vi "Overlays.vi"(0 "Image In":T2, 5 "FullArray":dbl[][](array[numeric]), 7 "SelectedGoalSubarray":dbl[](array[numeric]), 9 "ProjectedPosition":cluster{dbl, dbl}, 11 "Enabled Overlay":T3, 13 "Pitch":T1) -> (4 "Image Out":T2)   [LabVIEW 2012]
uses:
  <vilib>/vision/Image Controls.llb/IMAQ Image.ctl
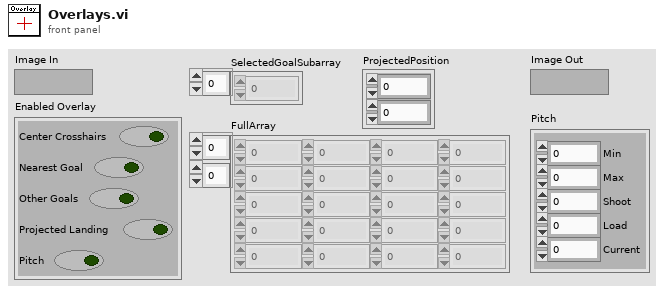
[diagram p1: front panel]
types:
  T1 = cluster{"Min":dbl, "Max":dbl, "Shoot":dbl, "Load":dbl, "Current":dbl}
  T2 = typedef "IMAQ Image.ctl" = refnum<image>
  T3 = cluster{"Center Crosshairs":bool, "Nearest Goal":bool, "Other Goals":bool, "Projected Landing":bool, "Pitch":bool}
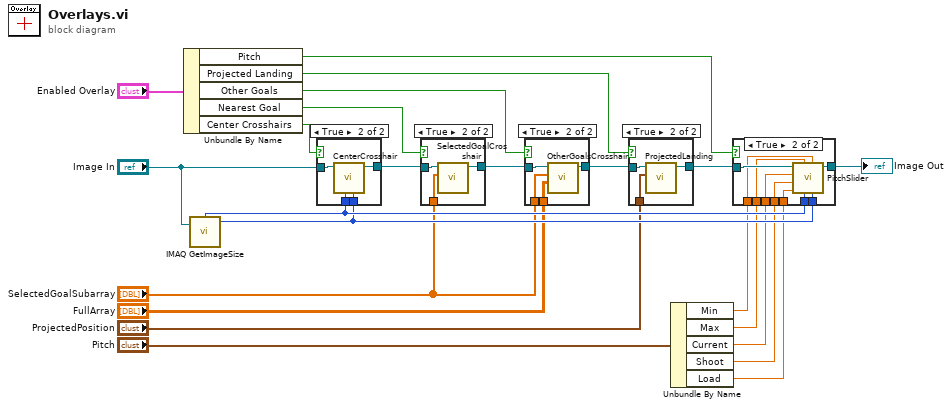
[diagram p0: block diagram]
diagram:
  n1 = Unbundle By Name("Enabled Overlay") -> ("Pitch"=w16:bool, "Projected Landing"=w17:bool, "Other Goals"=w18:bool, "Nearest Goal"=w20:bool, "Center Crosshairs"=w22:bool)
  n2 = call "IMAQ GetImageSize"("Image"="Image In") -> ("Y Resolution"=w10:i32, "X Resolution"=w11:i32)  [unwired: 3 in, 1 out]
  n3 = case shown="True" w22 {
    tunnel: "Image In" -> [w24 w28]
    tunnel: [w24 w27] -> w21
    tunnel: w11 -> [_ w26]
    tunnel: w10 -> [_ w25]
    frame False {
    }
    frame True {
      n4 = call "CenterCrosshair.vi"("Y Resolution"=w25, "X Resolution"=w26, "Image In"=w28) -> ("Image Out"=w27:T2)  [unwired: 8 in]
    }
  }
  n5 = case shown="True" w20 {
    tunnel: w21 -> [w29 w32]
    tunnel: [w29 w31] -> w15
    tunnel: "SelectedGoalSubarray" -> [_ w30]
    frame False {
    }
    frame True {
      n6 = call "SelectedGoalCrosshair.vi"("SelectedGoalSubarray"=w30, "Image In"=w32) -> ("Image Out"=w31:T2)  [unwired: 9 in]
    }
  }
  n7 = case shown="True" w18 {
    tunnel: w15 -> [w33 w37]
    tunnel: [w33 w36] -> w14
    tunnel: "FullArray" -> [_ w35]
    tunnel: "SelectedGoalSubarray" -> [_ w34]
    frame False {
    }
    frame True {
      n8 = call "OtherGoalsCrosshair.vi"("FullArray"=w35, "SelectedGoalSubarray"=w34, "Image In"=w37) -> ("Image Out"=w36:T2)  [unwired: 8 in]
    }
  }
  n9 = case shown="True" w17 {
    tunnel: w14 -> [w38 w41]
    tunnel: [w38 w40] -> w13
    tunnel: "ProjectedPosition" -> [_ w39]
    frame False {
    }
    frame True {
      n10 = call "ProjectedLanding.vi"("ProjectedPosition"=w39, "Image In"=w41) -> ("Image Out"=w40:T2)  [unwired: 9 in]
    }
  }
  n11 = Unbundle By Name("Pitch") -> ("Min"=w5:dbl, "Max"=w4:dbl, "Current"=w3:dbl, "Shoot"=w2:dbl, "Load"=w1:dbl)
  n12 = case shown="True" w16 {
    tunnel: w13 -> [w42 w51]
    tunnel: [w42 w50] -> w12
    tunnel: w11 -> [_ w49]
    tunnel: w10 -> [_ w48]
    tunnel: w5 -> [_ w43]
    tunnel: w4 -> [_ w44]
    tunnel: w3 -> [_ w45]
    tunnel: w2 -> [_ w46]
    tunnel: w1 -> [_ w47]
    frame False {
    }
    frame True {
      n13 = call "PitchSlider.vi"("Y Resolution"=w48, "Min"=w43, "X Resolution"=w49, "Max"=w44, "Load"=w47, "Shoot"=w46, "Current"=w45, "Image In"=w51) -> ("Image Out"=w50:T2)  [unwired: 3 in]
    }
  }
  "Image Out" <- w12
